vi "SalvaInDB.vi"(0 "CambiStato":T1[](array[typedef]), 1 "last":refnum<vi>) -> ()   [LabVIEW 2018]
uses:
  ControlConfigMisura.ctl
  ControlConfigDI.ctl
  D:/LIBRERIE_LV/SQLite/subvi/TypeDef/Tipo_sqlite_open.ctl
  D:/LIBRERIE_LV/SQLite/sqlite3.lvlib
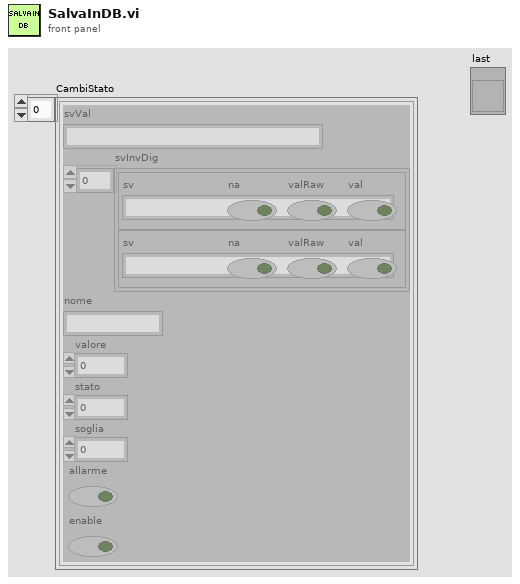
[diagram p1: front panel]
types:
  T1 = typedef "ControlConfigMisura.ctl" = cluster{"svVal":string, "svInvDig":T2[], "nome":string, "valore":dbl, "stato":i16, "soglia":dbl, "allarme":bool, "enable":bool}
  T2 = typedef "ControlConfigDI.ctl" = cluster{"sv":string, "na":bool, "valRaw":bool, "val":bool}
  T3 = typedef "sqlite3.lvlib/Tipo_sqlite_open.ctl" = enum16{"file", "in memory"}
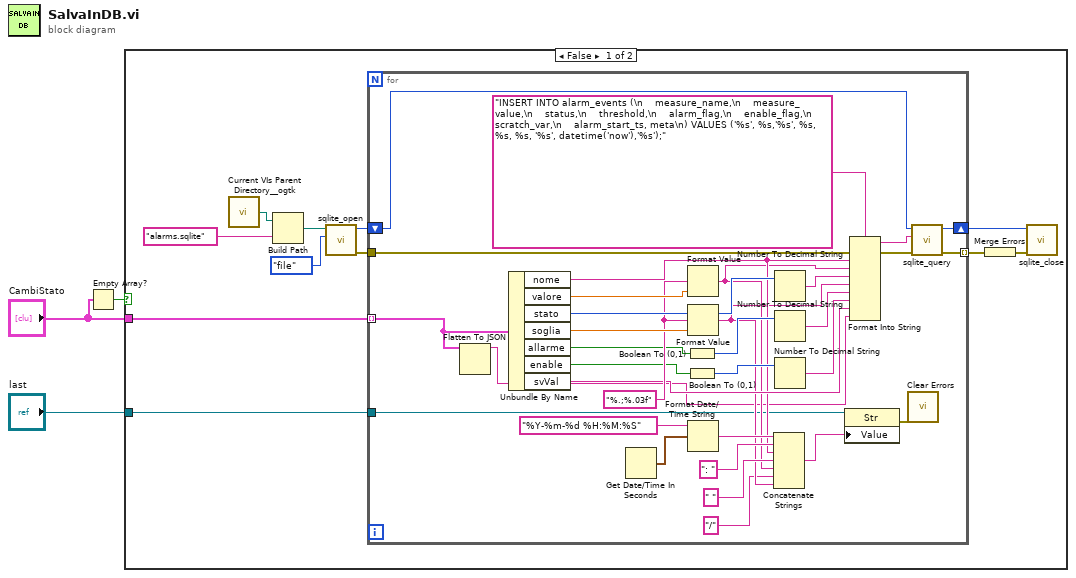
[diagram p0: block diagram]
diagram:
  n1 = Empty Array?(array="CambiStato") -> (empty?=w3:bool)
  n2 = case shown="False" w3 {
    tunnel: "CambiStato" -> [w8 _]
    tunnel: "last" -> [w4 _]
    frame False {
      n3 = call <userlib>:"Current VIs Parent Directory__ogtk.vi"() -> ("Parent Directory (+ Relative)"=w12:path)  [unwired: 5 in]
      n4 = Build Path(base path=w12, name or relative path="alarms.sqlite") -> (appended path=w11:path)
      n5 = call "sqlite_open.vi"("mode"=Tipo_sqlite_open."file", "Path"=w11) -> ("error out"=w5:errorcluster, "ppDb"=w14:u32)  [unwired: 8 in]
      n6 = for {
        shift-right: [w46] -> w13
        shift-left: w14 -> [w47]
        tunnel: w8 -> [w17] mode=indexing
        tunnel: [w31] -> w7 mode=indexing
        tunnel: w5 -> [w30]
        tunnel: w4 -> [w19]
        w40 = "%.;%.03f" ("format string")
        n7 = Flatten To JSON(anything=w17) -> (JSON string=w16:string)  [unwired: 2 in, 1 out]
        n8 = Unbundle By Name(w17) -> ("nome"=w24:string, "valore"=w42:dbl, "stato"=w44:i16, "soglia"=w41:dbl, "allarme"=w38:bool, "enable"=w35:bool, "svVal"=w33:string)
        n9 = Get Date/Time In Seconds() -> (seconds since 1Jan1904=w28:timestamp)
        n10 = Boolean To (0,1)(Boolean=w38) -> (0, 1=w39:i16)
        n11 = Boolean To (0,1)(Boolean=w35) -> (0, 1=w36:i16)
        n12 = Format Value(format string=w40, value (0)=w42) -> (output string=w22:string)  [unwired: 1 in]
        n13 = Format Value(format string=w40, value (0)=w41) -> (output string=w21:string)  [unwired: 1 in]
        n14 = Format Date/Time String(time format string (%c)="%Y-%m-%d %H:%M:%S", seconds (now)=w28) -> (date/time string=w26:string)  [unwired: 1 in]
        n15 = Concatenate Strings(w26, ": " ("string"), w24, " " ("string"), w22, "/" ("string"), w21) -> (w18:string)
        n16 = Number To Decimal String(number=w44) -> (decimal integer string=w43:string)  [unwired: 1 in]
        n17 = Number To Decimal String(number=w39) -> (decimal integer string=w37:string)  [unwired: 1 in]
        n18 = Number To Decimal String(number=w36) -> (decimal integer string=w34:string)  [unwired: 1 in]
        n19 = property class="Str"(reference=w19, "Value"=w18) -> (error out=w15:errorcluster)  [unwired: 1 in, 1 out]
        n20 = Format Into String(format string="INSERT INTO alarm_events (\n    measure_name,\n    measure_value,\n    status,\n    threshold,\n    alarm_flag,\n    enable_flag,\n    scratch_var,\n    alarm_start_ts, meta\n) VALUES ('%s', %s,'%s', %s, %s, %s, '%s', datetime('now'),'%s');", error in=w30, w24, w22, w43, w21, w37, w34, w33, w16) -> (resulting string=w32:string, error out=w29:errorcluster)  [unwired: 1 in]
        n21 = call <vilib>:"Clear Errors.vi"("error in (no error)"=w15) -> ()  [unwired: 5 in, 2 out]
        n22 = call "sqlite_query.vi"("error in (no error)"=w29, "Query"=w32, "db in"=w47) -> ("error out"=w31:errorcluster, "db out"=w46:u32)  [unwired: 6 in, 1 out]
      }
      n23 = Merge Errors(w7) -> (w6:errorcluster)
      n24 = call "sqlite_close.vi"("error in (no error)"=w6, "db in"=w13) -> ()  [unwired: 9 in, 1 out]
    }
    frame True {
    }
  }
